vi "New Stainless Correction Pop Up 2016.vi"(8 "error in (no error)":errorcluster, 9 "New Feet\n of Stainless\n(Count)":i32, 11 "Depth to \nWater Table\nInput":dbl) -> (0 "error in (no error) 2":errorcluster, 1 "Feet of\nStainless to be\nUsed (Count)":i32, 3 "Depth to \nWater Table\nOutput":dbl)   [LabVIEW 2016]
doc: "This vi allows the clinician to input the starting flexion. It used in order to derive a flexion correction."
uses:
  KPRO_lv2015/Kpro Globals.vi
panel:
  out "Original Feet\n of Stainless\n(Count)":i32
  in  "stop":bool
  in  "Increment Stainless":bool
  in  "Stainless OK As Is":bool
  in  "Correct Stainless":bool
  # "Please Choose \nto Correct, Increment, or to \nLeave Feet of Stainless as is"
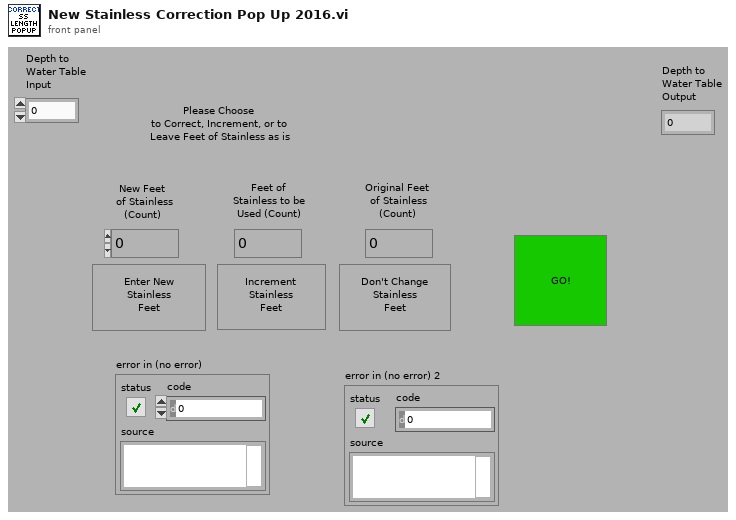
[diagram p1: front panel]
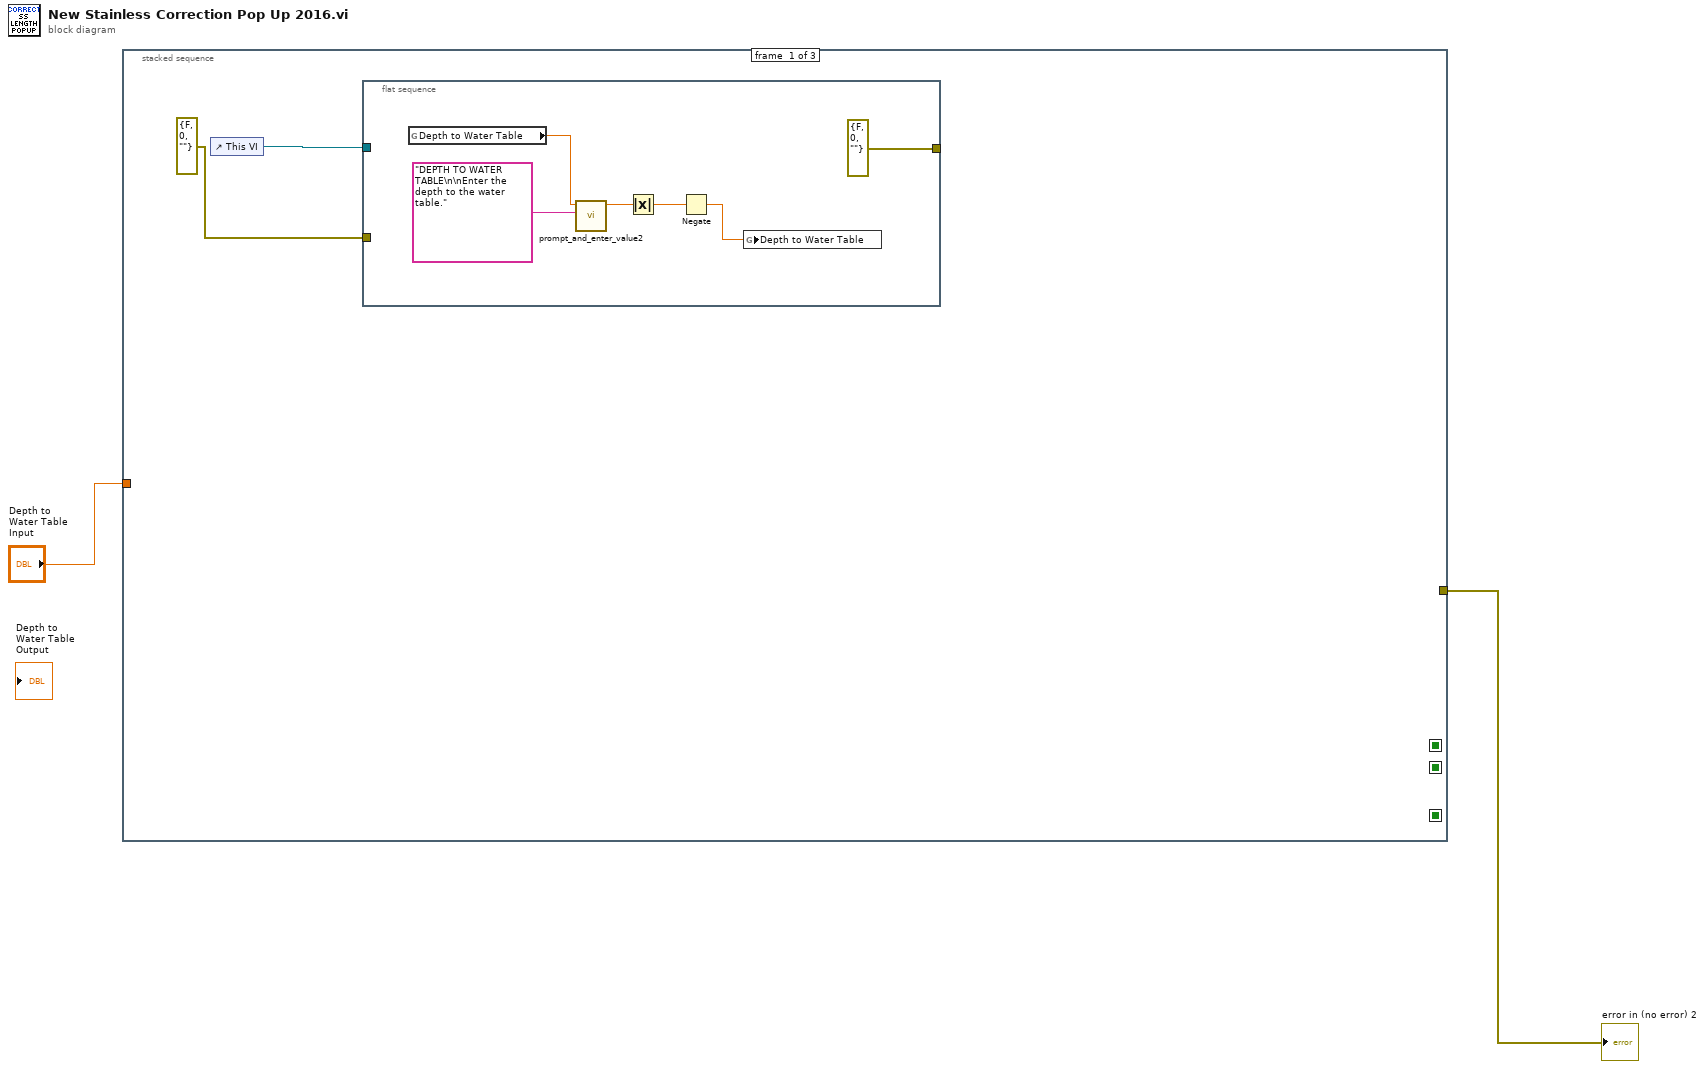
[diagram p0: block diagram]
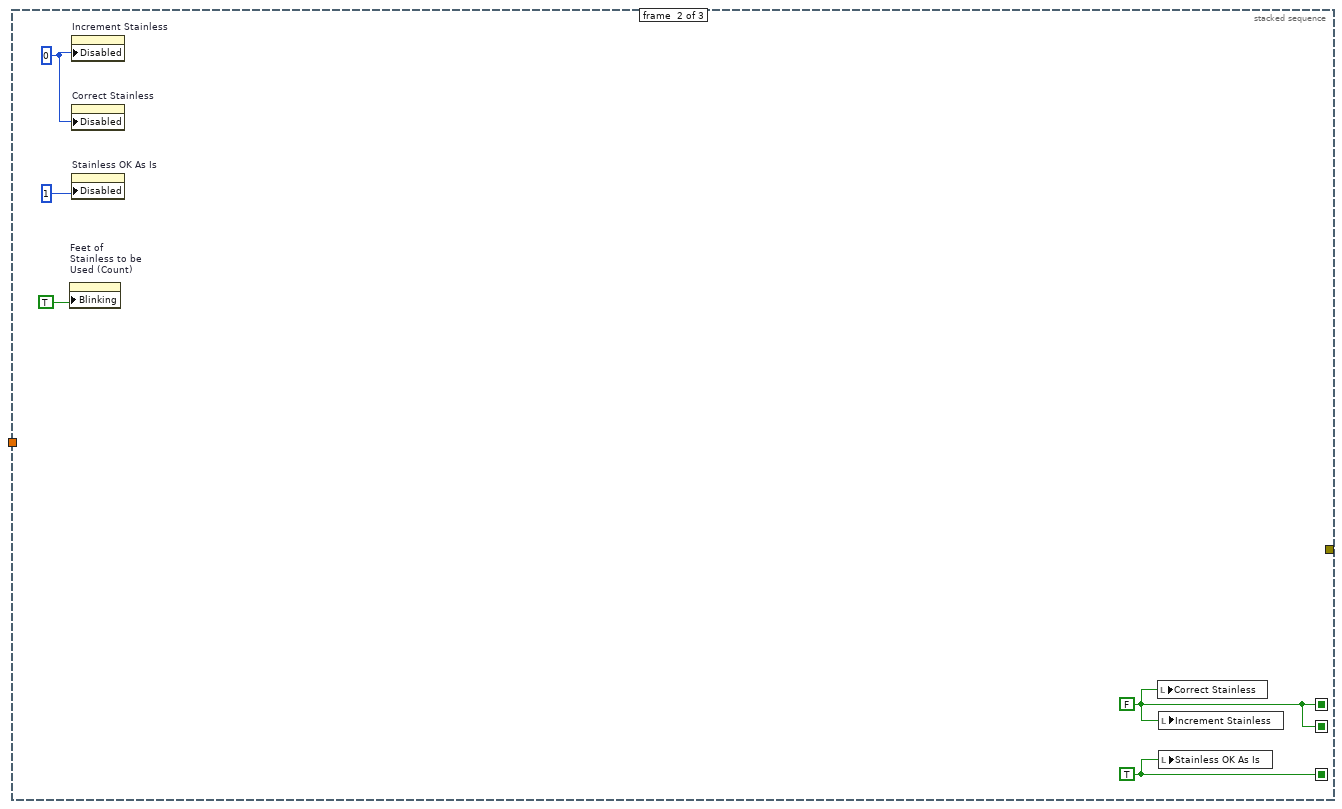
[diagram p2: hidden frame]
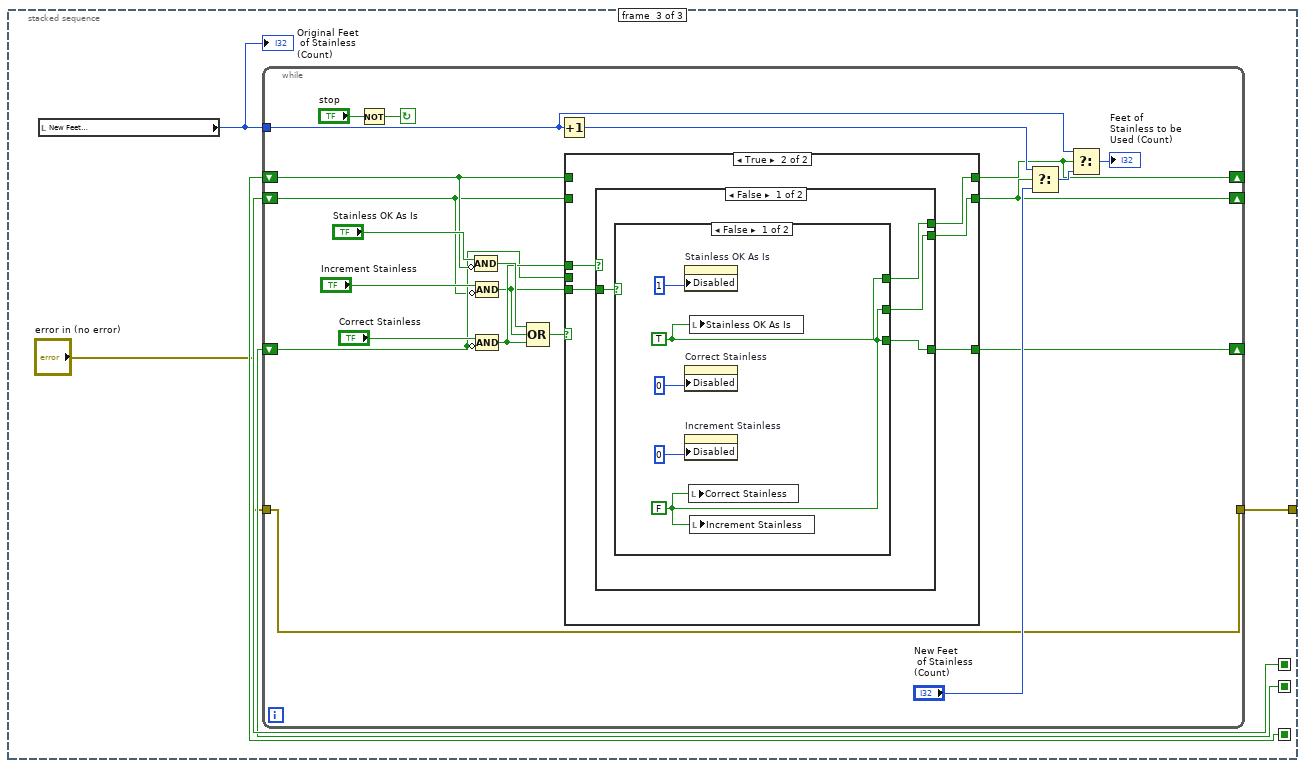
[diagram p3: hidden frame]
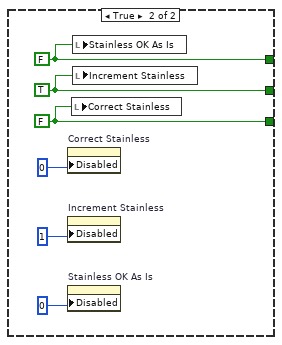
[diagram p5: hidden frame]
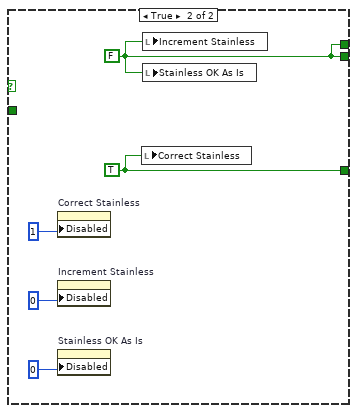
[diagram p6: hidden frame]
diagram:
  n1 = stacked-sequence {
    seq-local: [_ w14 _] -> [_ _ w19]
    seq-local: [_ w14 _] -> [_ _ w20]
    seq-local: [_ w15 _] -> [_ _ w21]
    tunnel: "Depth to \nWater Table\nInput" -> [_ _ _]
    tunnel: [_ _ w16] -> w1
    frame #0 {
      n2 = control-ref of="This VI"() -> (w4:refnum<vi>)
      n3 = flat-sequence {
        tunnel: [errorcluster {"status"=FALSE, "code"=0, "source"=""} ("error constant")] -> _
        tunnel: w4 -> [_]
        tunnel: errorcluster {"status"=FALSE, "code"=0, "source"=""} ("error constant") -> [_]
        frame #0 {
          n4 = global read "Kpro Globals.vi" "Depth to Water Table"() -> (w10:dbl)
          n5 = call "prompt_and_enter_value2.vi"("prompt_IN"="DEPTH TO WATER TABLE\n\nEnter the depth to the water table." ("prompt"), "Enter value"=w10) -> ("Numeric"=w6:dbl)  [unwired: 9 in]
          n6 = Absolute Value(x=w6) -> (abs(x)=w7:dbl)
          n7 = Negate(x=w7) -> (-x=w8:dbl)
          n8 = global write "Kpro Globals.vi" "Depth to Water Table"(w8) -> ()
        }
      }
    }
    frame #1 {
      w12 = 0
      w15 = TRUE
      w14 = FALSE
      n9 = property on="Feet of\nStainless to be\nUsed (Count)" class="DigNum (strict)"("Blinking"=TRUE) -> ()  [unwired: 2 in, 2 out]
      n10 = property on="Increment Stainless" class="Bool (strict)"("Disabled"=w12) -> ()  [unwired: 2 in, 2 out]
      n11 = property on="Correct Stainless" class="Bool (strict)"("Disabled"=w12) -> ()  [unwired: 2 in, 2 out]
      n12 = property on="Stainless OK As Is" class="Bool (strict)"("Disabled"=1) -> ()  [unwired: 2 in, 2 out]
      n13 = local write "Correct Stainless"(w14) -> ()
      n14 = local write "Increment Stainless"(w14) -> ()
      n15 = local write "Stainless OK As Is"(w15) -> ()
    }
    frame #2 {
      n16 = local read "New Feet\n of Stainless\n(Count)"() -> (w18:i32)
      "Original Feet\n of Stainless\n(Count)" <- w18
      n17 = while {
        tunnel: w18 -> [w24]
        shift-left: w19 -> [w26]
        shift-right: [w31] -> _
        shift-left: w20 -> [w25]
        shift-right: [w32] -> _
        shift-left: w21 -> [w27]
        shift-right: [w23] -> _
        tunnel: "error in (no error)" -> [w22]
        tunnel: [w22] -> w16
        stop <- w28 continue-if-true
        n18 = Not(x="stop") -> (.not. x?=w28:bool)
        n19 = Compound Arithmetic op=AND("Stainless OK As Is", invert w27) -> (w34:bool)
        n20 = Compound Arithmetic op=AND("Increment Stainless", invert w25) -> (w29:bool)
        n21 = Compound Arithmetic op=AND("Correct Stainless", invert w26) -> (w30:bool)
        n22 = Compound Arithmetic op=OR(w34, w29, w30) -> (w33:bool)
        n23 = Increment(x=w24) -> (x+1=w41:i32)
        n24 = case shown="True" w33 {
          tunnel: [w45 w48] -> w23
          tunnel: [w44 w47] -> w32
          tunnel: [w43 w49] -> w31
          tunnel: w30 -> [_ w50]
          tunnel: w29 -> [_ w46]
          tunnel: w27 -> [w45 _]
          tunnel: w26 -> [w43 _]
          tunnel: w25 -> [w44 _]
          frame False {
          }
          frame True {
            n25 = case shown="False" w50 {
              tunnel: [w51 w70] -> w49
              tunnel: [w53 w69] -> w48
              tunnel: [w52 w69] -> w47
              tunnel: w46 -> [w54 _]
              frame False {
                n26 = case shown="False" w54 {
                  tunnel: [w58 w63] -> w53
                  tunnel: [w59 w64] -> w52
                  tunnel: [w59 w65] -> w51
                  frame False {
                    w58 = TRUE
                    w59 = FALSE
                    n27 = property on="Stainless OK As Is" class="Bool (strict)"("Disabled"=1) -> ()  [unwired: 2 in, 2 out]
                    n28 = property on="Correct Stainless" class="Bool (strict)"("Disabled"=0) -> ()  [unwired: 2 in, 2 out]
                    n29 = property on="Increment Stainless" class="Bool (strict)"("Disabled"=0) -> ()  [unwired: 2 in, 2 out]
                    n30 = local write "Correct Stainless"(w59) -> ()
                    n31 = local write "Stainless OK As Is"(w58) -> ()
                    n32 = local write "Increment Stainless"(w59) -> ()
                  }
                  frame True {
                    w63 = FALSE
                    w64 = TRUE
                    w65 = FALSE
                    n33 = property on="Correct Stainless" class="Bool (strict)"("Disabled"=0) -> ()  [unwired: 2 in, 2 out]
                    n34 = property on="Increment Stainless" class="Bool (strict)"("Disabled"=1) -> ()  [unwired: 2 in, 2 out]
                    n35 = property on="Stainless OK As Is" class="Bool (strict)"("Disabled"=0) -> ()  [unwired: 2 in, 2 out]
                    n36 = local write "Correct Stainless"(w65) -> ()
                    n37 = local write "Stainless OK As Is"(w63) -> ()
                    n38 = local write "Increment Stainless"(w64) -> ()
                  }
                }
              }
              frame True {
                w69 = FALSE
                w70 = TRUE
                n39 = property on="Correct Stainless" class="Bool (strict)"("Disabled"=1) -> ()  [unwired: 2 in, 2 out]
                n40 = property on="Increment Stainless" class="Bool (strict)"("Disabled"=0) -> ()  [unwired: 2 in, 2 out]
                n41 = property on="Stainless OK As Is" class="Bool (strict)"("Disabled"=0) -> ()  [unwired: 2 in, 2 out]
                n42 = local write "Correct Stainless"(w70) -> ()
                n43 = local write "Increment Stainless"(w69) -> ()
                n44 = local write "Stainless OK As Is"(w69) -> ()
              }
            }
          }
        }
        n45 = Select(t=w41, s=w32, f="New Feet\n of Stainless\n(Count)") -> (s? t:f=w40:i32)
        n46 = Select(t=w24, s=w23, f=w40) -> (s? t:f=→"Feet of\nStainless to be\nUsed (Count)":i32)
      }
    }
  }
  "error in (no error) 2" <- w1
